vi "Move_LDA_Mirror_Low.vi"(3 "Mode":T1, 4 "Extra Commands":string, 5 "Mirror Up?":bool=TRUE) -> (0 "Error Message":string, 1 "Initially Mirror Up?":bool)   [LabVIEW 2020]
uses:
  Controls/User_Specific_mode.ctl
  Controls/Tunnel_Coordinates.ctl
  Trav_mode.ctl
  Globals/Preference_global.vi
  Globals/Constants_global.vi
  Globals/Trav_pos_global.vi
  Route mapping/Route_mapping_global.vi
  Collision_Detection/Triangles/EnFlo specific/Collision Detection global.vi
panel:
  out "Current Traverse Position":sgl[](array[numeric]) format="%#.2f"
  out "Start Traverse Position":sgl[](array[numeric]) format="%#.2f"
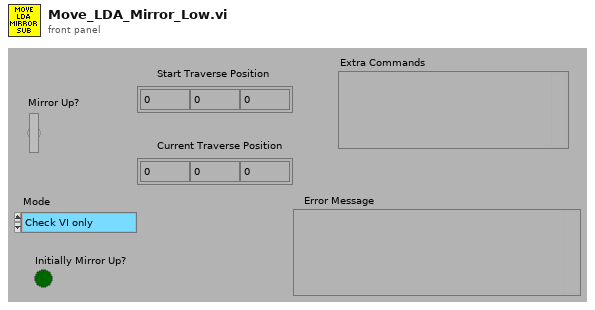
[diagram p1: front panel]
types:
  T1 = typedef "User_Specific_mode.ctl" = enum16{"Check VI only", "Run VI"}
  T2 = typedef "Tunnel_Coordinates.ctl" = enum16{"Work in Tunnel Coordinates", "Work in Model Coordinates"}
  T3 = typedef "Trav_mode.ctl" = enum16{"Move traverse", "Read traverse position", "Teach Position"}
  T4 = typedef "Box_size.ctl" = cluster{"Max":sgl, "Min":sgl}[]
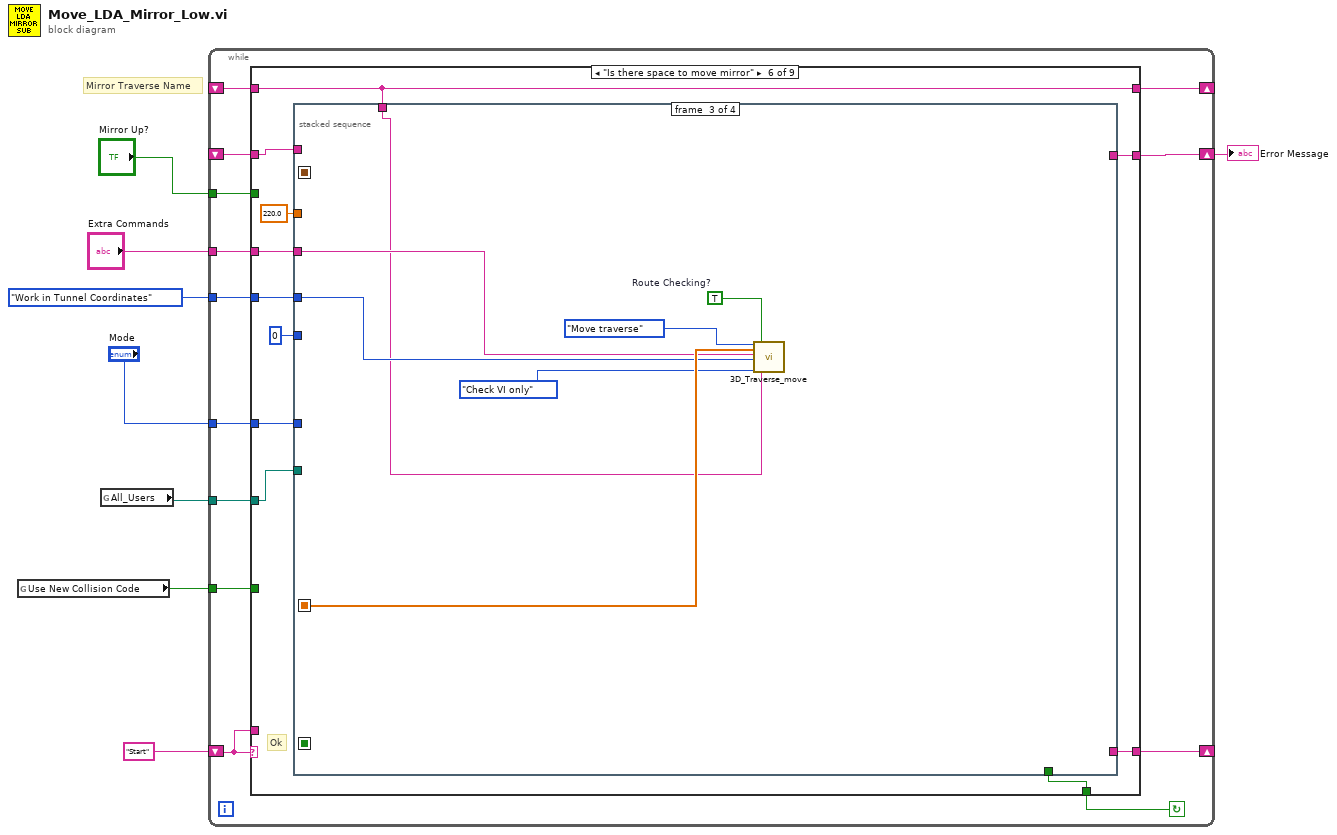
[diagram p0: block diagram]
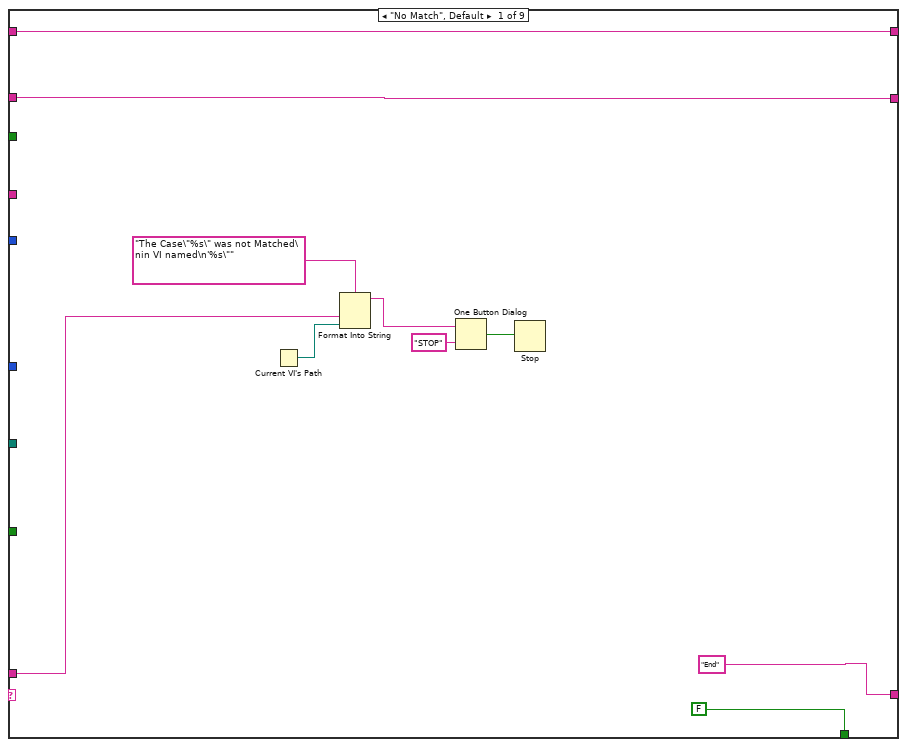
[diagram p2: hidden frame]
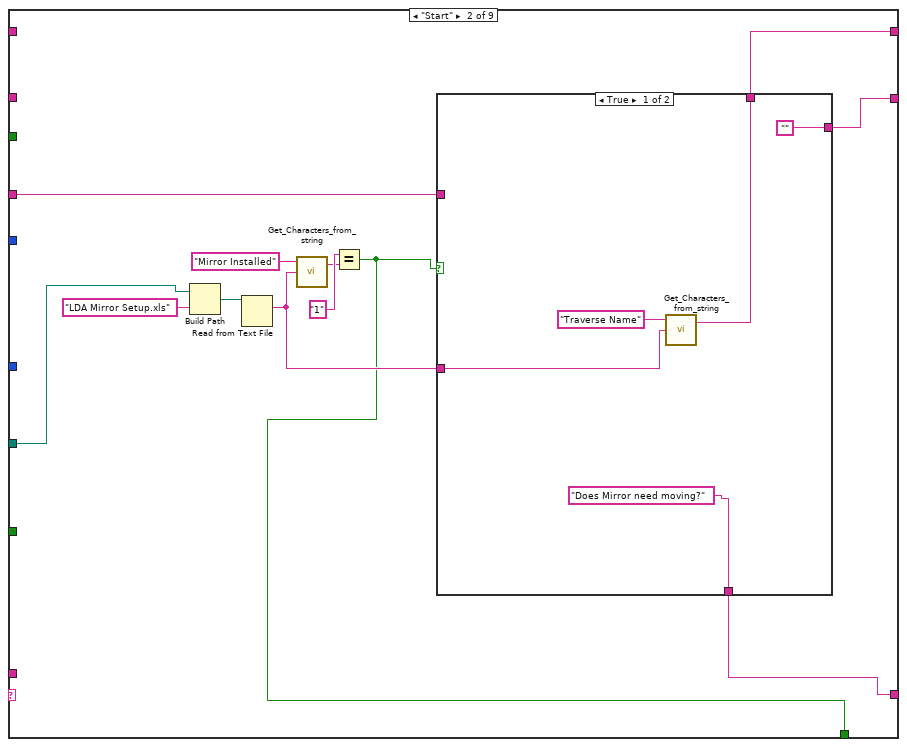
[diagram p3: hidden frame]
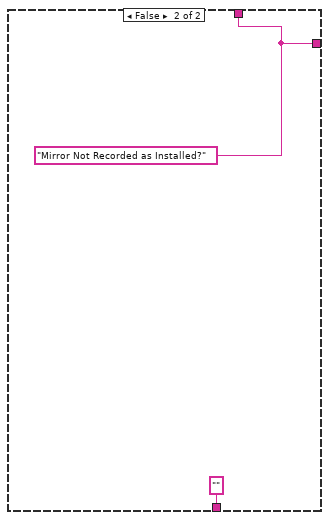
[diagram p4: hidden frame]
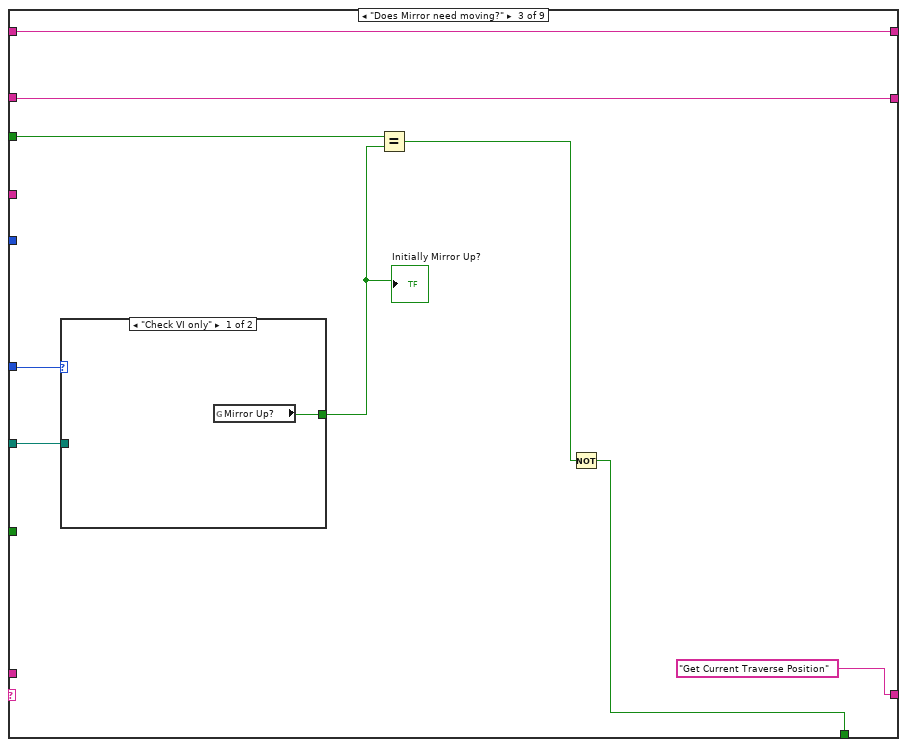
[diagram p5: hidden frame]
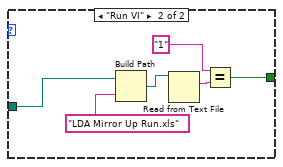
[diagram p6: hidden frame]
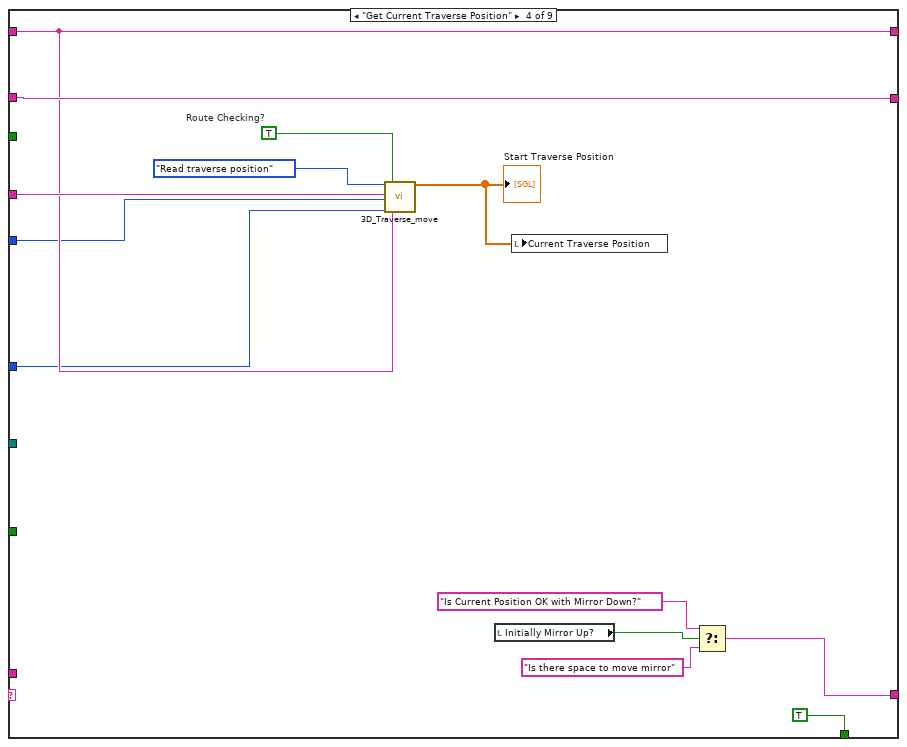
[diagram p7: hidden frame]
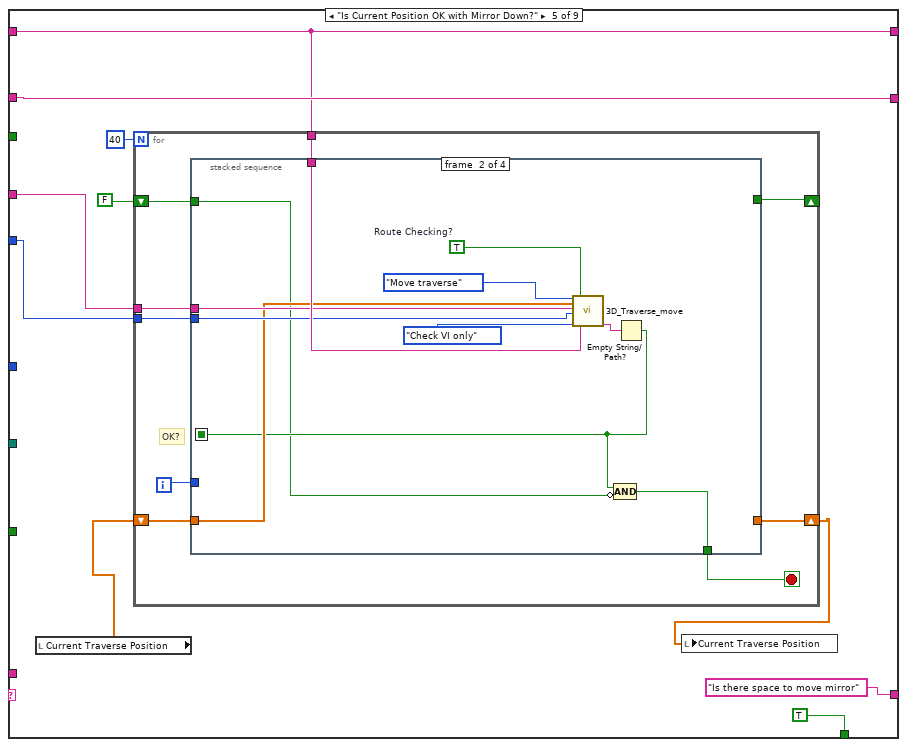
[diagram p8: hidden frame]
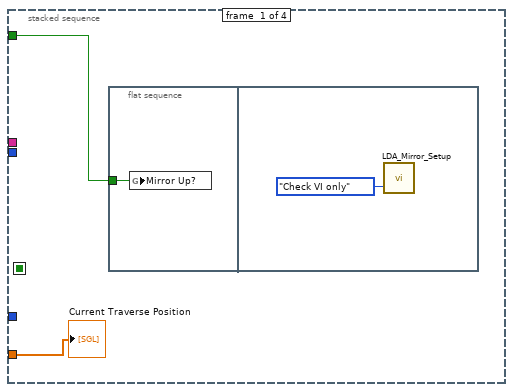
[diagram p9: hidden frame]
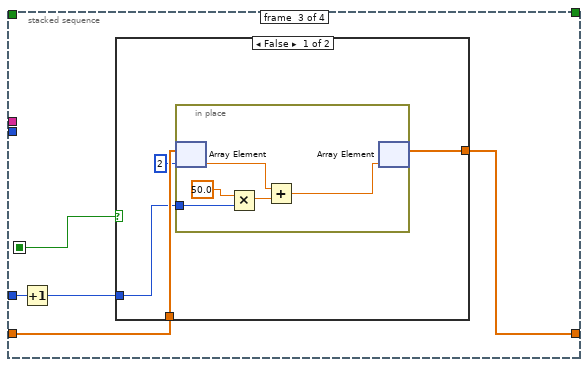
[diagram p10: hidden frame]
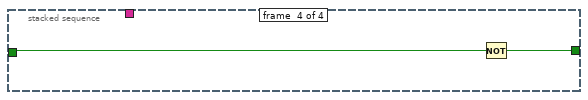
[diagram p12: hidden frame]
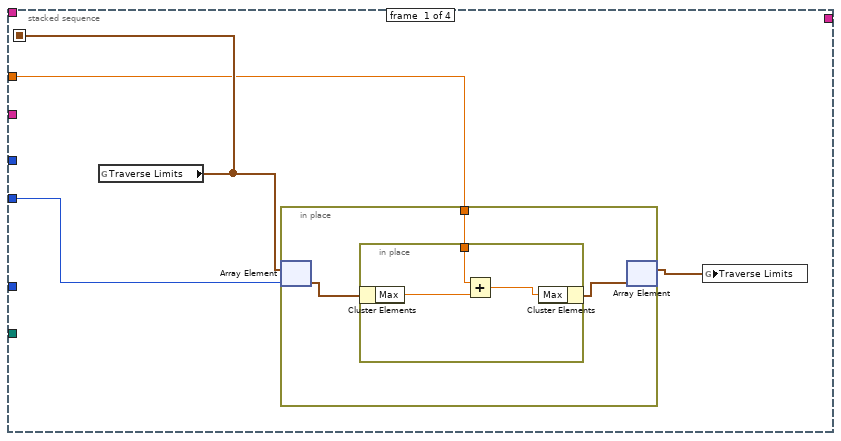
[diagram p13: hidden frame]
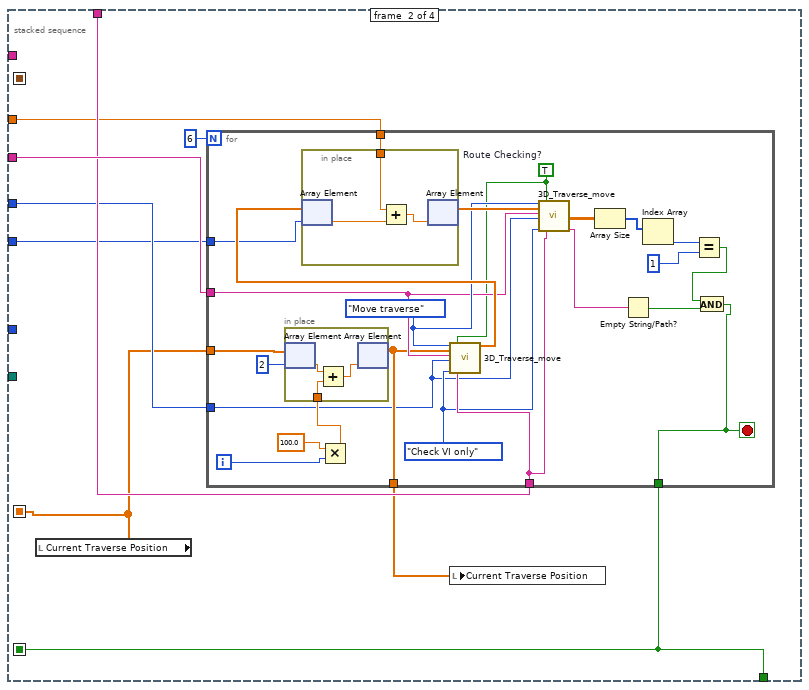
[diagram p14: hidden frame]
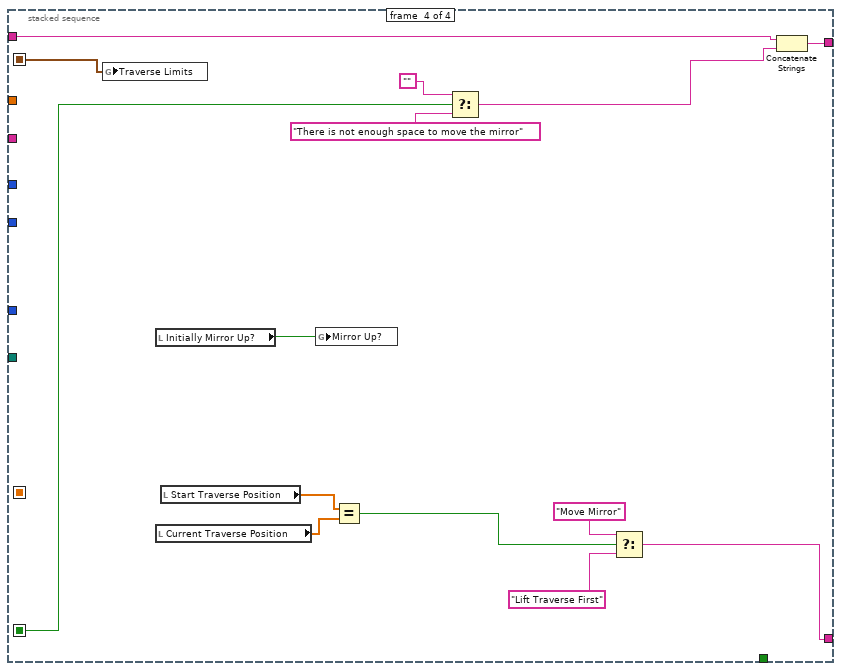
[diagram p15: hidden frame]
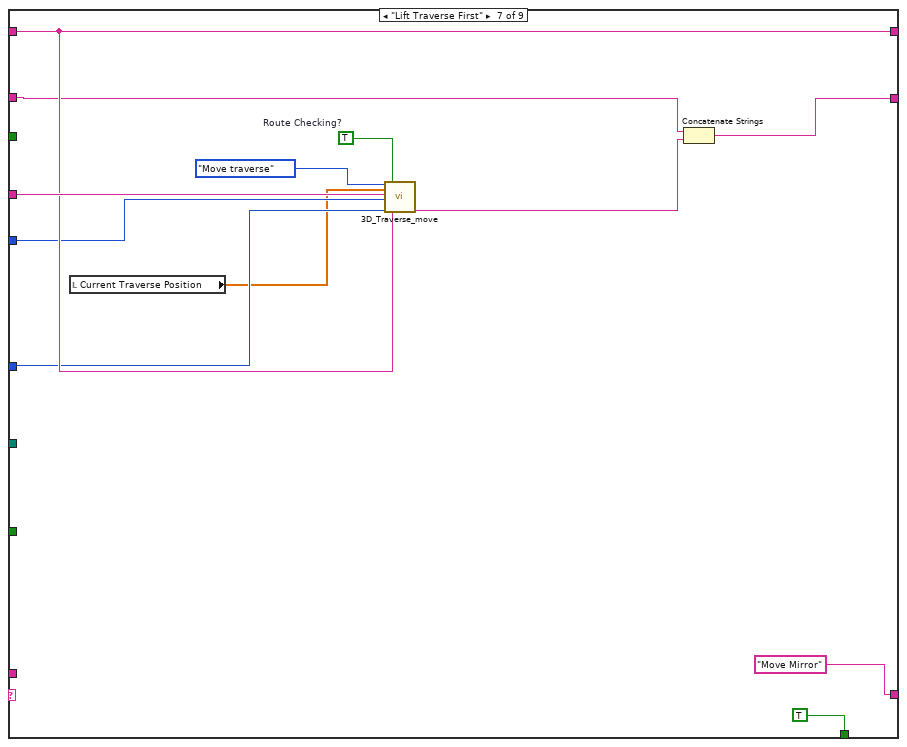
[diagram p16: hidden frame]
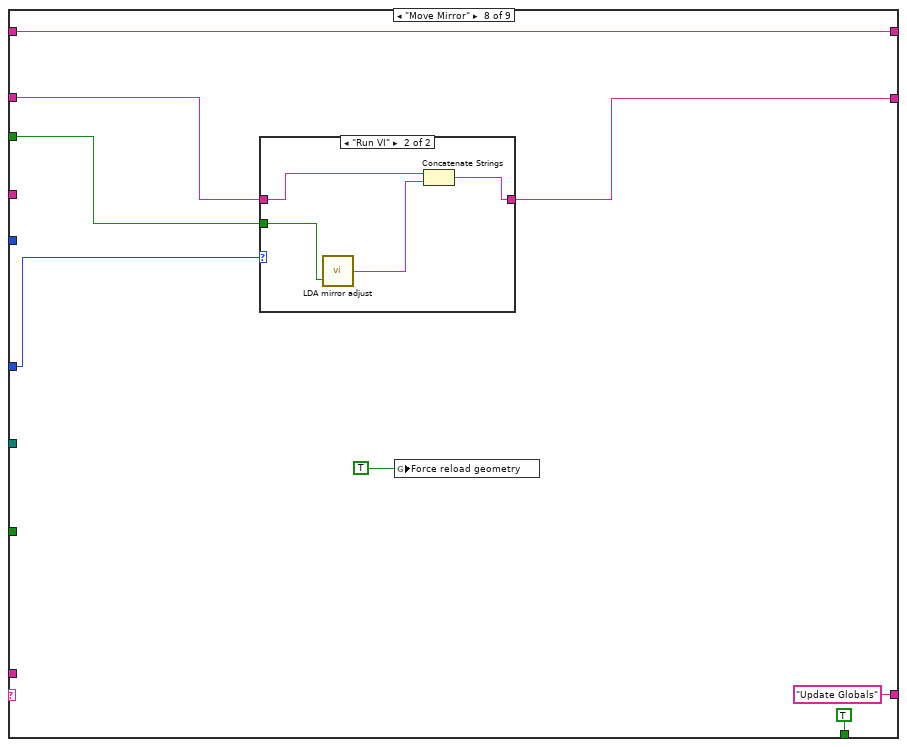
[diagram p17: hidden frame]
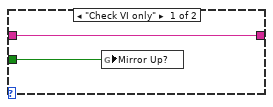
[diagram p18: hidden frame]
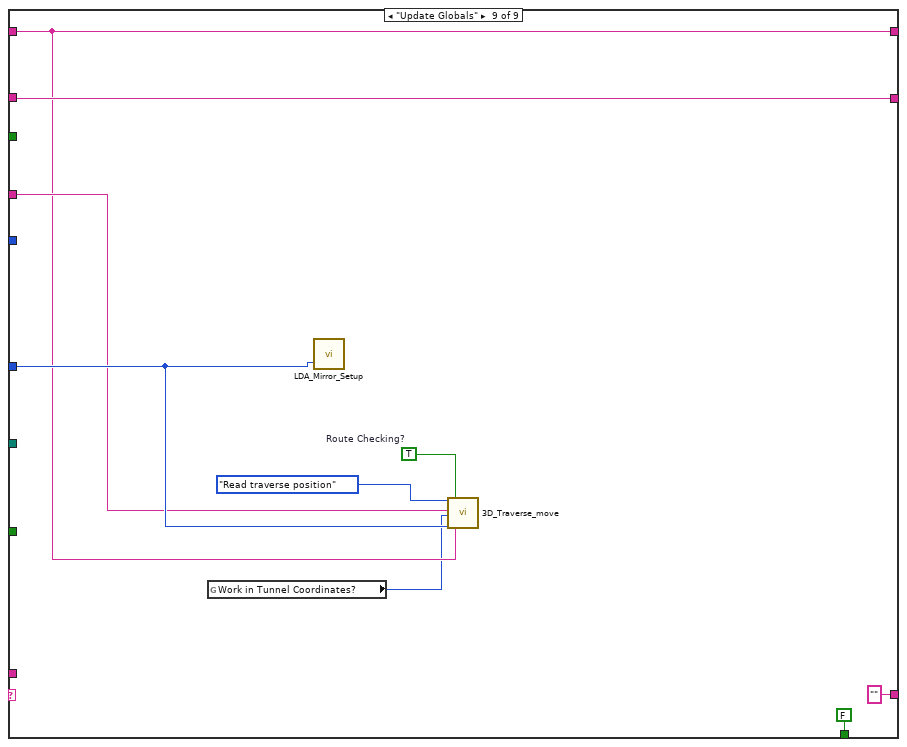
[diagram p19: hidden frame]
diagram:
  # "Mirror Traverse Name"
  n1 = global read "Preference_global.vi" "Use New Collision Code"() -> (w4:bool)
  n2 = global read "Constants_global.vi" "All_Users"() -> (w3:path)
  n3 = while {
    shift-left: _ -> [w19]
    shift-right: [w17] -> w6
    tunnel: "Mode" -> [w21]
    shift-left: "Start" -> [w18]
    shift-right: [w20] -> _
    shift-right: [w16] -> _
    shift-left: _ -> [w14]
    tunnel: "Extra Commands" -> [w15]
    tunnel: w4 -> [w12]
    tunnel: w3 -> [w11]
    tunnel: "Mirror Up?" -> [w10]
    tunnel: Tunnel_Coordinates."Work in Tunnel Coordinates" ("Work in Tunnel Coordinates") -> [w9]
    stop <- w13 continue-if-true
    n4 = case shown="\"Is there space to move mirror\"" w18 {
      tunnel: w21 -> [_ _ w54 w67 _ w136 w216 w231 w241]
      tunnel: ["End" w40 "Get Current Traverse Position" w68 "Is there space to move mirror" w141 "Move Mirror" "Update Globals" ""] -> w20
      tunnel: w19 -> [w26 _ w57 w79 w88 w138 w214 w224 w246]
      tunnel: [w26 w43 w57 w79 w88 w137 w212 w229 w246] -> w17
      tunnel: w18 -> [w24 _ _ _ _ _ _ _ _]
      tunnel: [w23 w42 w58 w74 w85 w139 w219 w230 w239] -> w16
      tunnel: w15 -> [_ w41 _ w75 w86 w140 w220 _ w240]
      tunnel: w14 -> [w23 _ w58 w74 w85 w139 w219 w230 w239]
      tunnel: [FALSE ("Update Datum Powers?") w32 w56 TRUE ("Update Datum Powers?") TRUE ("Update Datum Powers?") w135 TRUE ("Update Datum Powers?") TRUE ("Update Datum Powers?") FALSE ("Update Datum Powers?")] -> w13
      tunnel: w12 -> [_ _ _ _ _ _ _ _ _]
      tunnel: w11 -> [_ w33 w55 _ _ w134 _ _ _]
      tunnel: w10 -> [_ _ w53 _ _ _ _ w225 _]
      tunnel: w9 -> [_ _ _ w73 w84 w133 w218 _ _]
      frame "No Match", Default {
        n5 = Current VI's Path() -> (path=w27:path)
        n6 = Format Into String(format string="The Case\"%s\" was not Matched\nin VI named\n'%s\"" ("Format String"), w24, w27) -> (resulting string=w30:string)  [unwired: 2 in, 1 out]
        n7 = One Button Dialog(message=w30, button name ("OK")="STOP") -> (true=w28:bool)
        n8 = Stop(stop? (T)=w28) -> ()
      }
      frame "Start" {
        n9 = Build Path(base path=w33, name or relative path="LDA Mirror Setup.xls") -> (appended path=w37:path)
        n10 = Read from Text File(file (use dialog)=w37) -> (text=w34:string)  [unwired: 3 in, 3 out]
        n11 = call "Get_Characters_from_string.vi"("Input string"=w34, "Variable name"="Mirror Installed") -> ("Value"=w38:string)  [unwired: 1 in, 1 out]
        n12 = Equal?(x="1" ("String to match"), y=w38) -> (x = y?=w32:bool)
        n13 = case shown="True" w32 {
          tunnel: ["" w50] -> w43
          tunnel: [w45 w50] -> w42
          tunnel: w41 -> [_ _]
          tunnel: ["Does Mirror need moving?" ""] -> w40
          tunnel: w34 -> [w44 _]
          frame True {
            n14 = call "Get_Characters_from_string.vi"("Input string"=w44, "Variable name"="Traverse Name") -> ("Value"=w45:string)  [unwired: 1 in, 1 out]
          }
          frame False {
            w50 = "Mirror Not Recorded as Installed?"
          }
        }
      }
      frame "Does Mirror need moving?" {
        n15 = case shown="\"Check VI only\"" w54 {
          tunnel: w55 -> [_ w63]
          tunnel: [w60 w61] -> w52
          frame "Check VI only" {
            n16 = global read "Trav_pos_global.vi" "Mirror Up?"() -> (w60:bool)
          }
          frame "Run VI" {
            n17 = Build Path(base path=w63, name or relative path="LDA Mirror Up Run.xls") -> (appended path=w64:path)
            n18 = Read from Text File(file (use dialog)=w64) -> (text=w65:string)  [unwired: 3 in, 3 out]
            n19 = Equal?(x="1" ("String to match"), y=w65) -> (x = y?=w61:bool)
          }
        }
        "Initially Mirror Up?" <- w52
        n20 = Equal?(x=w53, y=w52) -> (x = y?=w59:bool)
        n21 = Not(x=w59) -> (.not. x?=w56:bool)
      }
      frame "Get Current Traverse Position" {
        w76 = TRUE  # Route Checking?
        n22 = call "3D_Traverse_move.vi"("Mode"=Trav_mode."Read traverse position", "Extra command String"=w75, "Work in Tunnel Coordinates"=w73, "Simulate/Run"=w67, "Route Checking?"=w76, "Traverse name"=w74) -> ("Trav Position achieved"=w69:sgl[])  [unwired: 10 in, 3 out]
        "Start Traverse Position" <- w69
        n23 = local read "Initially Mirror Up?"() -> (w70:bool)
        n24 = local write "Current Traverse Position"(w69) -> ()
        n25 = Select(t="Is Current Position OK with Mirror Down?", s=w70, f="Is there space to move mirror") -> (s? t:f=w68:string)
      }
      frame "Is Current Position OK with Mirror Down?" {
        n26 = local read "Current Traverse Position"() -> (w80:sgl[])
        n27 = for {
          N: 40 -> [_]
          tunnel: w86 -> [w98]
          tunnel: w85 -> [w97]
          tunnel: w84 -> [w96]
          shift-right: [w92] -> w81
          shift-left: w80 -> [w94]
          shift-right: [w90] -> _
          shift-left: FALSE -> [w95]
          i -> [w93]
          stop <- w91 stop-if-true
          # "OK?"
          n28 = stacked-sequence {
            seq-local: [_ w105 _ _] -> [_ _ w114 _]
            tunnel: w98 -> [_ w108 _ _]
            tunnel: w96 -> [_ w109 _ _]
            tunnel: w97 -> [_ w110 _ _]
            tunnel: w95 -> [w100 w104 _ w130]
            tunnel: w94 -> [w99 w107 w116 _]
            tunnel: w93 -> [_ _ w118 _]
            tunnel: [_ _ w115 _] -> w92
            tunnel: [_ w103 _ _] -> w91
            tunnel: [_ _ _ w129] -> w90
            frame #0 {
              n29 = flat-sequence {
                tunnel: w100 -> [w101]
                frame #0 {
                  n30 = global write "Trav_pos_global.vi" "Mirror Up?"(w101) -> ()
                }
                frame #1 {
                  n31 = call "LDA_Mirror_Setup.vi"("Simulate/Run"=User_Specific_mode."Check VI only") -> ()  [unwired: 3 in, 1 out]
                }
              }
              "Current Traverse Position" <- w99
            }
            frame #1 {
              w111 = TRUE  # Route Checking?
              n32 = call "3D_Traverse_move.vi"("Mode"=Trav_mode."Move traverse", "Position"=w107, "Extra command String"=w108, "Work in Tunnel Coordinates"=w109, "Simulate/Run"=User_Specific_mode."Check VI only", "Route Checking?"=w111, "Traverse name"=w110) -> ("Error String"=w106:string)  [unwired: 9 in, 3 out]
              n33 = Empty String/Path?(string/path=w106) -> (empty?=w105:bool)
              n34 = Compound Arithmetic op=AND(w105, invert w104) -> (w103:bool)
            }
            frame #2 {
              n35 = Increment(x=w118) -> (x+1=w117:i32)
              n36 = case shown="False" w114 {
                tunnel: w117 -> [w120 _]
                tunnel: w116 -> [w122 w128]
                tunnel: [w119 w128] -> w115
                frame False {
                  n37 = in-place {
                    in-place-border: w120 -> [w127]
                    n38 = in-place-array #1(w122, 2) -> (w124:sgl)
                    n39 = Multiply(x=sgl 50.0, y=w127) -> (x*y=w125:sgl)
                    n40 = Add(x=w124, y=w125) -> (x+y=w123:sgl)
                    n41 = in-place-array #1(w123) -> (w119:sgl[])  [unwired: 1 out]
                  }
                }
                frame True {
                }
              }
            }
            frame #3 {
              n42 = Not(x=w130) -> (.not. x?=w129:bool)
            }
          }
        }
        n43 = local write "Current Traverse Position"(w81) -> ()
      }
      frame "Is there space to move mirror" {
        # "Ok"
        n44 = stacked-sequence {
          seq-local: [_ w156 _ _] -> [_ _ _ w206]
          seq-local: [w145 _ _ _] -> [_ _ _ w198]
          seq-local: [_ w152 _ _] -> [_ _ w195 _]
          tunnel: [_ _ _ w200] -> w141
          tunnel: w140 -> [_ w159 w194 _]
          tunnel: w139 -> [_ w158 w191 _]
          tunnel: w138 -> [_ _ _ w209]
          tunnel: [_ _ _ w207] -> w137
          tunnel: w136 -> [_ _ _ _]
          tunnel: [_ w156 _ _] -> w135
          tunnel: w134 -> [_ _ _ _]
          tunnel: w133 -> [_ w155 w193 _]
          tunnel: sgl 220.0 ("x") -> [w144 w154 _ _]
          tunnel: 0 -> [w142 w153 _ _]
          frame #0 {
            n45 = global read "Route_mapping_global.vi" "Traverse Limits"() -> (w145:T4)
            n46 = in-place {
              in-place-border: w144 -> [w147]
              n47 = in-place-array #2(w145, w142) -> (w148:cluster{"Max":sgl, "Min":sgl})
              n48 = in-place {
                in-place-border: w147 -> [w150]
                n49 = in-place-cluster #3(w148) -> ("Max"=w151:sgl)
                n50 = Add(x=w150, y=w151) -> (x+y=w149:sgl)
                n51 = in-place-cluster #3("Max"=w149) -> (w146:cluster{"Max":sgl, "Min":sgl})
              }
              n52 = in-place-array #2(w146) -> (w143:T4)  [unwired: 1 out]
            }
            n53 = global write "Route_mapping_global.vi" "Traverse Limits"(w143) -> ()
          }
          frame #1 {
            n54 = local read "Current Traverse Position"() -> (w152:sgl[])
            n55 = for {
              N: 6 -> [_]
              tunnel: w158 -> [w176]
              tunnel: w159 -> [w177]
              tunnel: w152 -> [w181]
              tunnel: [w165] -> w157
              tunnel: [w166] -> w156
              tunnel: w155 -> [w163]
              tunnel: w154 -> [w162]
              tunnel: w153 -> [w161]
              i -> [w167]
              stop <- w166 stop-if-true
              w164 = TRUE  # Route Checking?
              w178 = Trav_mode."Move traverse" ("Mode")
              w175 = User_Specific_mode."Check VI only" ("Simulate/Run")
              n56 = Multiply(x=sgl 100.0, y=w167) -> (x*y=w182:sgl)
              n57 = in-place {
                in-place-border: w182 -> [w189]
                n58 = in-place-array #4(w181, 2) -> (w190:sgl)
                n59 = Add(x=w190, y=w189) -> (x+y=w188:sgl)
                n60 = in-place-array #4(w188) -> (w165:sgl[])  [unwired: 1 out]
              }
              n61 = call "3D_Traverse_move.vi"("Mode"=w178, "Position"=w165, "Extra command String"=w177, "Work in Tunnel Coordinates"=w163, "Simulate/Run"=w175, "Route Checking?"=w164, "Traverse name"=w176) -> ("Trav Position achieved"=w180:sgl[])  [unwired: 9 in, 3 out]
              n62 = in-place {
                in-place-border: w162 -> [w185]
                n63 = in-place-array #5(w180, w161) -> (w187:sgl)
                n64 = Add(x=w185, y=w187) -> (x+y=w186:sgl)
                n65 = in-place-array #5(w186) -> (w179:sgl[])  [unwired: 1 out]
              }
              n66 = call "3D_Traverse_move.vi"("Mode"=w178, "Position"=w179, "Extra command String"=w177, "Work in Tunnel Coordinates"=w163, "Simulate/Run"=w175, "Route Checking?"=w164, "Traverse name"=w176) -> ("Valid Steps before Trav to Trav (Tun Cord)"=w173:sgl[][], "Error String"=w174:string)  [unwired: 9 in, 2 out]
              n67 = Array Size(array=w173) -> (size(s)=w172:i32[])
              n68 = Empty String/Path?(string/path=w174) -> (empty?=w169:bool)
              n69 = Index Array(array=w172) -> (element=w171:i32)  [unwired: 1 in]
              n70 = Equal?(x=w171, y=1) -> (x = y?=w168:bool)
              n71 = And(x=w168, y=w169) -> (x .and. y?=w166:bool)
            }
            n72 = local write "Current Traverse Position"(w157) -> ()
          }
          frame #2 {
            w196 = TRUE  # Route Checking?
            n73 = call "3D_Traverse_move.vi"("Mode"=Trav_mode."Move traverse", "Position"=w195, "Extra command String"=w194, "Work in Tunnel Coordinates"=w193, "Simulate/Run"=User_Specific_mode."Check VI only", "Route Checking?"=w196, "Traverse name"=w191) -> ()  [unwired: 9 in, 4 out]
          }
          frame #3 {
            n74 = global write "Route_mapping_global.vi" "Traverse Limits"(w198) -> ()
            n75 = local read "Initially Mirror Up?"() -> (w199:bool)
            n76 = local read "Current Traverse Position"() -> (w205:sgl[])
            n77 = local read "Start Traverse Position"() -> (w204:sgl[])
            n78 = global write "Trav_pos_global.vi" "Mirror Up?"(w199) -> ()
            n79 = Equal?(x=w204, y=w205) -> (x = y?=w203:bool)
            n80 = Select(t="", s=w206, f="There is not enough space to move the mirror") -> (s? t:f=w208:string)
            n81 = Select(t="Move Mirror", s=w203, f="Lift Traverse First") -> (s? t:f=w200:string)
            n82 = Concatenate Strings(w209, w208) -> (w207:string)
          }
        }
      }
      frame "Lift Traverse First" {
        w221 = TRUE  # Route Checking?
        n83 = local read "Current Traverse Position"() -> (w215:sgl[])
        n84 = call "3D_Traverse_move.vi"("Mode"=Trav_mode."Move traverse", "Position"=w215, "Extra command String"=w220, "Work in Tunnel Coordinates"=w218, "Simulate/Run"=w216, "Route Checking?"=w221, "Traverse name"=w219) -> ("Error String"=w213:string)  [unwired: 9 in, 3 out]
        n85 = Concatenate Strings(w214, w213) -> (w212:string)
      }
      frame "Move Mirror" {
        n86 = case shown="\"Run VI\"" w231 {
          tunnel: [w232 w235] -> w229
          tunnel: w225 -> [w233 w234]
          tunnel: w224 -> [w232 w236]
          frame "Check VI only" {
            n87 = global write "Trav_pos_global.vi" "Mirror Up?"(w233) -> ()
          }
          frame "Run VI" {
            n88 = call "LDA mirror adjust.vi"("Mirror Up?"=w234) -> ("Error String"=w237:string)  [unwired: 1 in]
            n89 = Concatenate Strings(w236, w237) -> (w235:string)
          }
        }
        n90 = global write "Collision Detection global.vi" "Force reload geometry"(TRUE ("Reload geometry")) -> ()
      }
      frame "Update Globals" {
        w242 = TRUE  # Route Checking?
        n91 = global read "Trav_pos_global.vi" "Work in Tunnel Coordinates?"() -> (w238:T2)
        n92 = call "LDA_Mirror_Setup.vi"("Simulate/Run"=w241) -> ()  [unwired: 3 in, 1 out]
        n93 = call "3D_Traverse_move.vi"("Mode"=Trav_mode."Read traverse position", "Extra command String"=w240, "Work in Tunnel Coordinates"=w238, "Simulate/Run"=w241, "Route Checking?"=w242, "Traverse name"=w239) -> ()  [unwired: 10 in, 4 out]
      }
    }
  }
  "Error Message" <- w6
